vi "tsdb_get_lin_db_signal_properties_by_index.vi"(4 "FIsTx":u8, 6 "FSignalIndex":i32, 7 "FFrameIndex":i32, 8 "error in (no error)":errorcluster caption="错误输入（无错误）", 9 "FECUIndex":i32, 10 "FDBIndex":i32, 11 "路径输入":path=path "D:/Program Files (x86)/TOSUN/TSMaster/bin/TSMaster.dll") -> (0 "error out":errorcluster caption="错误输出", 1 "TDBSignalProperties":T1, 2 "function return":i32, 3 "路径输出":path)   [LabVIEW 2014]
doc: "Function Introduction\nRetrieve the signal attributes of the specified LIN database through frame index\nCall location\ninput parameter \nAIdxDB: Database Index\nFrameIdx: database frame index\nAIndes: signal index in frame\nAvalue: The returned attribute data structure, please search for the definition in the TSMaster header\nReturn value\n==0: Execution successful\nOther values: Query error code"
uses:
  Typedef/CAN/TCANSignal.ctl
  Typedef/LIN/TLINSignal.ctl
  Typedef/FlexRay/TFlexRaySignal.ctl
  Typedef/TDBSignalProperties.ctl
panel:
  # "typedef enum _TSignalType {stCANSignal, stLINSignal, stSystemVar, stFlexRay, stEthernet} TSignalType;"
  # "typedef struct _TCANSignal{\n    u8     FCANSgnType; // 0 - Unsigned, 1 - Signed, 2 - Single 32, 3 - Double 64\n    bool   FIsIntel;\n    s32    FStartBit;\n    s32    FLength;    \n    double FFactor;\n    double FOffset;    \n} TCANSignal, *PCANSignal;\n// LIN signal record, size = 26\ntypedef struct _TLINSignal{\n    u8     FLINSgnType; // 0 - Unsigned, 1 - Signed, 2 - Single 32, 3 - Double 64\n    bool   FIsIntel;\n    s32    FStartBit;\n    s32    FLength;    \n    double FFactor;\n    double FOffset;    \n} TLINSignal, *PLINSignal;\n// FlexRay signal record, size = 32\ntypedef struct _TFlexRaySignal{\n    u8     FFRSgnType;   // 0 - Unsigned, 1 - Signed, 2 - Single 32, 3 - Double 64\n    u8     FCompuMethod; // 0 - Identical, 1 - Linear, 2 - Scale Linear, 3 - TextTable, 4 - TABNoIntp, 5 - Formula\n    u8     FReserved;\n    bool   FIsIntel;\n    s32    FStartBit;\n    s32    FUpdateBit;\n    s32    FLength;\n    double FFactor;\n    double FOffset;\n    s32    FActualStartBit;\n    s32    FActualUpdateBit;\n} TFlexRaySignal, *PFlexRaySignal;"
  # "typedef struct _TDBSignalProperties {\n    s32 FDBIndex;\n    s32 FECUIndex;\n    s32 FFrameIndex;\n    s32 FSignalIndex;\n    u8  FIsTx;    \n    u8  FReserved1;\n    u8  FReserved2;\n    u8  FReserved3;\n    TSignalType    FSignalType;    \n    TCANSignal     FCANSignal;\n    TLINSignal     FLINSignal;\n    TFlexRaySignal FFlexRaySignal;\n    s32            FParentFrameId;\n    double         FInitValue;\n    char FName[DATABASE_STR_LEN];\n    char FComment[DATABASE_STR_LEN];\n} TDBSignalProperties, *PDBSignalProperties;"
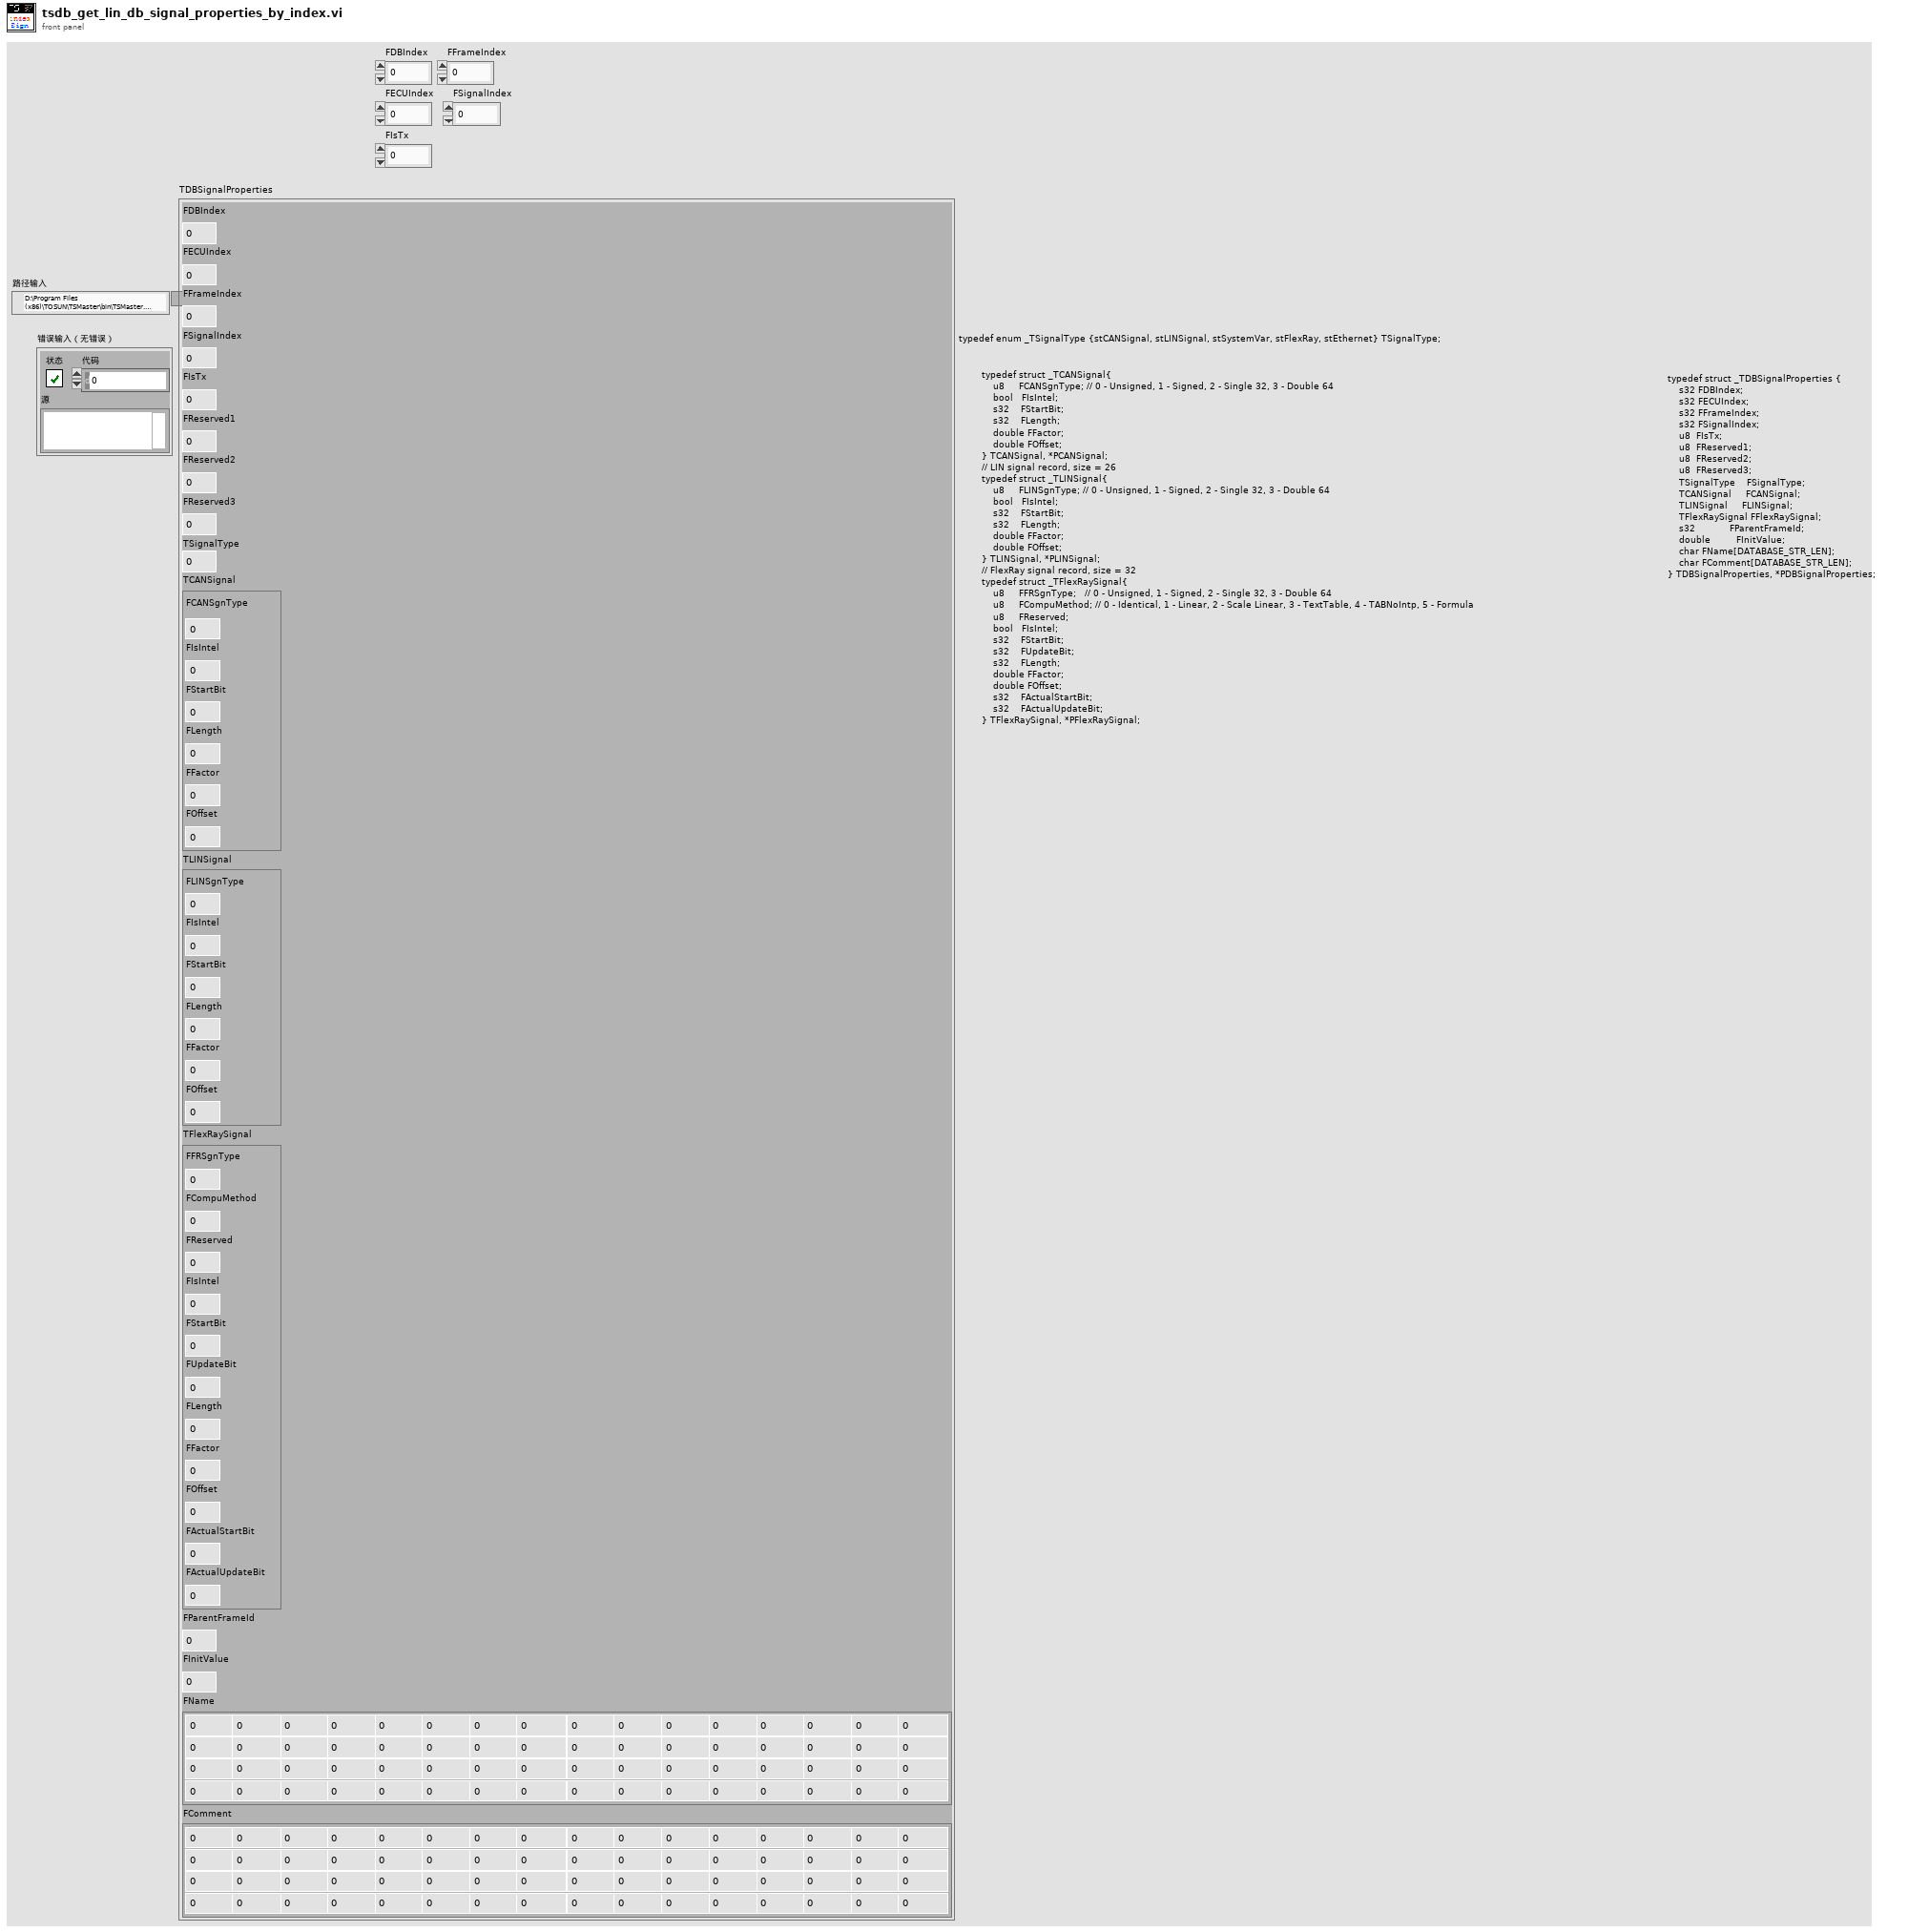
[diagram p1: front panel]
types:
  T1 = typedef "TDBSignalProperties.ctl" = cluster{"FDBIndex":i32, "FECUIndex":i32, "FFrameIndex":i32, "FSignalIndex":i32, "FIsTx":u8, "FReserved1":u8, "FReserved2":u8, "FReserved3":u8, "TSignalType":i32, "TCANSignal":T2, "TLINSignal":T3, "TFlexRaySignal":T4, "FParentFrameId":i32, "FInitValue":dbl, "FName":cluster{"数值":u64, "数值 2":u64, "数值 3":u64, "数值 4":u64, "数值 5":u64, "数值 6":u64, "数值 7":u64, "数值 8":u64, "数值 9":u64, "数值 10":u64, "数值 11":u64, "数值 12":u64, "数值 13":u64, "数值 14":u64, "数值 15":u64, "数值 16":u64, "数值 17":u64, "数值 18":u64, "数值 19":u64, "数值 20":u64, "数值 21":u64, "数值 22":u64, "数值 23":u64, "数值 24":u64, "数值 25":u64, "数值 26":u64, "数值 27":u64, "数值 28":u64, "数值 29":u64, "数值 30":u64, "数值 31":u64, "数值 32":u64, "数值 33":u64, "数值 34":u64, "数值 35":u64, "数值 36":u64, "数值 37":u64, "数值 38":u64, "数值 39":u64, "数值 40":u64, "数值 41":u64, "数值 42":u64, "数值 43":u64, "数值 44":u64, "数值 45":u64, "数值 46":u64, "数值 47":u64, "数值 48":u64, "数值 49":u64, "数值 50":u64, "数值 51":u64, "数值 52":u64, "数值 53":u64, "数值 54":u64, "数值 55":u64, "数值 56":u64, "数值 57":u64, "数值 58":u64, "数值 59":u64, "数值 60":u64, "数值 61":u64, "数值 62":u64, "数值 63":u64, "数值 64":u64}, "FComment":cluster{"数值":u64, "数值 2":u64, "数值 3":u64, "数值 4":u64, "数值 5":u64, "数值 6":u64, "数值 7":u64, "数值 8":u64, "数值 9":u64, "数值 10":u64, "数值 11":u64, "数值 12":u64, "数值 13":u64, "数值 14":u64, "数值 15":u64, "数值 16":u64, "数值 17":u64, "数值 18":u64, "数值 19":u64, "数值 20":u64, "数值 21":u64, "数值 22":u64, "数值 23":u64, "数值 24":u64, "数值 25":u64, "数值 26":u64, "数值 27":u64, "数值 28":u64, "数值 29":u64, "数值 30":u64, "数值 31":u64, "数值 32":u64, "数值 33":u64, "数值 34":u64, "数值 35":u64, "数值 36":u64, "数值 37":u64, "数值 38":u64, "数值 39":u64, "数值 40":u64, "数值 41":u64, "数值 42":u64, "数值 43":u64, "数值 44":u64, "数值 45":u64, "数值 46":u64, "数值 47":u64, "数值 48":u64, "数值 49":u64, "数值 50":u64, "数值 51":u64, "数值 52":u64, "数值 53":u64, "数值 54":u64, "数值 55":u64, "数值 56":u64, "数值 57":u64, "数值 58":u64, "数值 59":u64, "数值 60":u64, "数值 61":u64, "数值 62":u64, "数值 63":u64, "数值 64":u64}}
  T2 = typedef "TCANSignal.ctl" = cluster{"FCANSgnType":u8, "FIsIntel":u8, "FStartBit":i32, "FLength":i32, "FFactor":dbl, "FOffset":dbl}
  T3 = typedef "TLINSignal.ctl" = cluster{"FLINSgnType":u8, "FIsIntel":u8, "FStartBit":i32, "FLength":i32, "FFactor":dbl, "FOffset":dbl}
  T4 = typedef "TFlexRaySignal.ctl" = cluster{"FFRSgnType":u8, "FCompuMethod":u8, "FReserved":u8, "FIsIntel":u8, "FStartBit":i32, "FUpdateBit":i32, "FLength":i32, "FFactor":dbl, "FOffset":dbl, "FActualStartBit":i32, "FActualUpdateBit":i32}
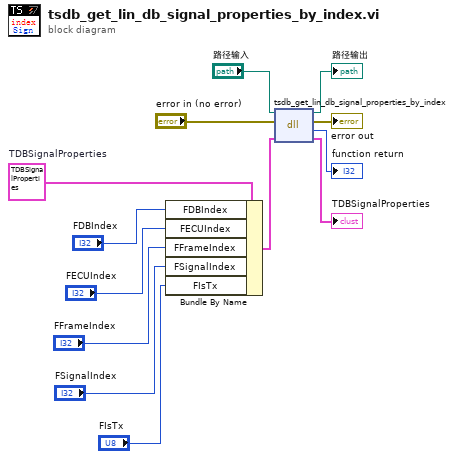
[diagram p0: block diagram]
diagram:
  w7 = T1 {"FDBIndex"=0, "FECUIndex"=0, "FFrameIndex"=0, "FSignalIndex"=0, "FIsTx"=0, "FReserved1"=0, "FReserved2"=0, "FReserved3"=0, "TSignalType"=0, "TCANSignal"={"FCANSgnType"=0, "FIsIntel"=0, "FStartBit"=0, "FLength"=0, "FFactor"=0.0, "FOffset"=0.0}, "TLINSignal"={"FLINSgnType"=0, "FIsIntel"=0, "FStartBit"=0, "FLength"=0, "FFactor"=0.0, "FOffset"=0.0}, "TFlexRaySignal"={"FFRSgnType"=0, "FCompuMethod"=0, "FReserved"=0, "FIsIntel"=0, "FStartBit"=0, "FUpdateBit"=0, "FLength"=0, "FFactor"=0.0, "FOffset"=0.0, "FActualStartBit"=0, "FActualUpdateBit"=0}, "FParentFrameId"=0, "FInitValue"=0.0, "FName"={"数值"=0, "数值 2"=0, "数值 3"=0, "数值 4"=0, "数值 5"=0, "数值 6"=0, "数值 7"=0, "数值 8"=0, "数值 9"=0, "数值 10"=0, "数值 11"=0, "数值 12"=0, "数值 13"=0, "数值 14"=0, "数值 15"=0, "数值 16"=0, "数值 17"=0, "数值 18"=0, "数值 19"=0, "数值 20"=0, "数值 21"=0, "数值 22"=0, "数值 23"=0, "数值 24"=0, "数值 25"=0, "数值 26"=0, "数值 27"=0, "数值 28"=0, "数值 29"=0, "数值 30"=0, "数值 31"=0, "数值 32"=0, "数值 33"=0, "数值 34"=0, "数值 35"=0, "数值 36"=0, "数值 37"=0, "数值 38"=0, "数值 39"=0, "数值 40"=0, "数值 41"=0, "数值 42"=0, "数值 43"=0, "数值 44"=0, "数值 45"=0, "数值 46"=0, "数值 47"=0, "数值 48"=0, "数值 49"=0, "数值 50"=0, "数值 51"=0, "数值 52"=0, "数值 53"=0, "数值 54"=0, "数值 55"=0, "数值 56"=0, "数值 57"=0, "数值 58"=0, "数值 59"=0, "数值 60"=0, "数值 61"=0, "数值 62"=0, "数值 63"=0, "数值 64"=0}, "FComment"={"数值"=0, "数值 2"=0, "数值 3"=0, "数值 4"=0, "数值 5"=0, "数值 6"=0, "数值 7"=0, "数值 8"=0, "数值 9"=0, "数值 10"=0, "数值 11"=0, "数值 12"=0, "数值 13"=0, "数值 14"=0, "数值 15"=0, "数值 16"=0, "数值 17"=0, "数值 18"=0, "数值 19"=0, "数值 20"=0, "数值 21"=0, "数值 22"=0, "数值 23"=0, "数值 24"=0, "数值 25"=0, "数值 26"=0, "数值 27"=0, "数值 28"=0, "数值 29"=0, "数值 30"=0, "数值 31"=0, "数值 32"=0, "数值 33"=0, "数值 34"=0, "数值 35"=0, "数值 36"=0, "数值 37"=0, "数值 38"=0, "数值 39"=0, "数值 40"=0, "数值 41"=0, "数值 42"=0, "数值 43"=0, "数值 44"=0, "数值 45"=0, "数值 46"=0, "数值 47"=0, "数值 48"=0, "数值 49"=0, "数值 50"=0, "数值 51"=0, "数值 52"=0, "数值 53"=0, "数值 54"=0, "数值 55"=0, "数值 56"=0, "数值 57"=0, "数值 58"=0, "数值 59"=0, "数值 60"=0, "数值 61"=0, "数值 62"=0, "数值 63"=0, "数值 64"=0}}  # TDBSignalProperties
  n1 = Bundle By Name(cluster=w7, "FDBIndex"="FDBIndex", "FECUIndex"="FECUIndex", "FFrameIndex"="FFrameIndex", "FSignalIndex"="FSignalIndex", "FIsTx"="FIsTx") -> (w6:T1)
  n2 = dll-call lib="D:/Work/LabVIEW Code/TSMaster Labview SDK/LabVIEW/LabVIEW-TSMasterAPI_CLN/TSMasterAPI_LabVIEW-2024-08-27 16-32-25/Not_organized_vi/TSMaster.*" fn="tsdb_get_lin_db_signal_properties_by_index"(path in="路径输入", error in="error in (no error)", "Avalue"=w6) -> (path out=→"路径输出":path, error out=→"error out":errorcluster, "返回类型"=→"function return":i32, "Avalue"=→"TDBSignalProperties":T1)  [unwired: 1 in]
